vi "Identify Contraction Segment.vi"(10 "Intra-cursor segment":dynamicdata(waveform), 11 "Contraction Onset":dbl) -> (1 "Con Ons on I-C Segment":dbl, 2 "Contraction Segment":dynamicdata(waveform), 3 "Con Ons Segment":dynamicdata(waveform), 4 "trigger location":dbl)   [LabVIEW 2016]
uses:
  <vilib>/measure/mamon.llb/Trigger Detection for 1 Channel.vi
  <vilib>/measure/NI_MAPro.lvlib
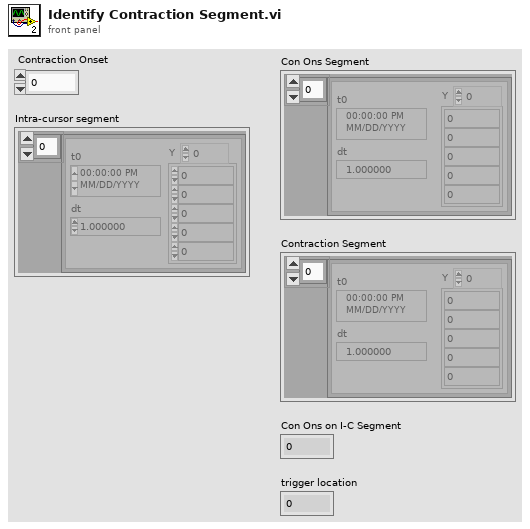
[diagram p1: front panel]
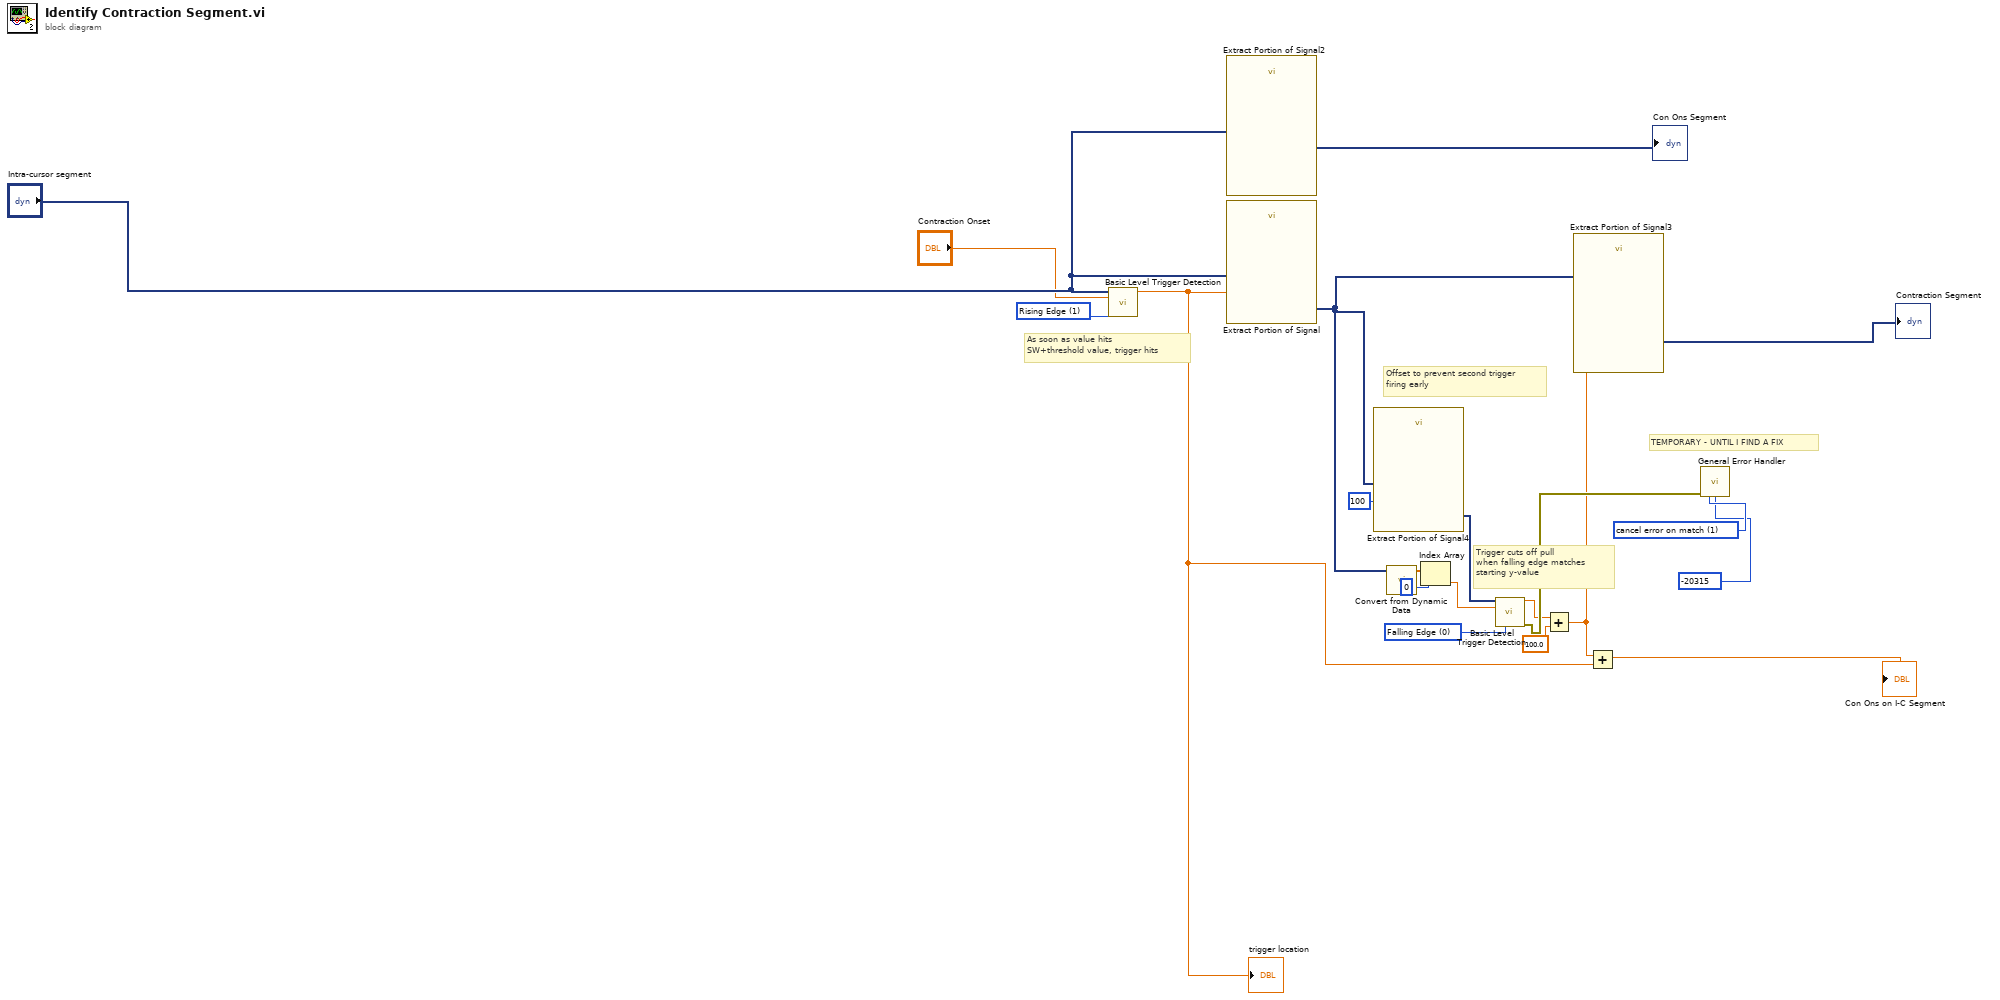
[diagram p0: block diagram]
diagram:
  w19 = 1 items=["no exception", "cancel error on match", "set error on match"] ("[exception action] (none:0)")
  w3 = u16 0 items=["Falling Edge", "Rising Edge"] ("trigger slope")
  w1 = u16 1 items=["Falling Edge", "Rising Edge"] ("trigger slope")
  # "TEMPORARY - UNTIL I FIND A FIX"
  # "Offset to prevent second trigger\nfiring early"
  # "Trigger cuts off pull\nwhen falling edge matches \nstarting y-value"
  # "As soon as value hits \nSW+threshold value, trigger hits"
  n1 = call-poly <vilib>:"Basic Level Trigger Detection.vi"("signal in"="Intra-cursor segment", "level"="Contraction Onset", "trigger slope"=w1) -> ("trigger location"=w11:dbl)  [unwired: 10 in, 2 out]
  "trigger location" <- w11
  n2 = call "Extract Portion of Signal2"("Signals"="Intra-cursor segment") -> ("Section"=→"Con Ons Segment":dynamicdata)  [unwired: 9 in, 1 out]
  n3 = call "Extract Portion of Signal"("Begin Sample"=w11, "Signals"="Intra-cursor segment") -> ("Section"=w12:dynamicdata)  [unwired: 8 in, 1 out]
  n4 = call "Extract Portion of Signal4"("Begin Sample"=100, "Signals"=w12) -> ("Section"=w14:dynamicdata)  [unwired: 8 in, 1 out]
  n5 = call "Convert from Dynamic Data"("Dynamic Data Type"=w12) -> ("Array"=w7:dbl[])  [unwired: 3 in]
  n6 = Index Array(array=w7, index=0) -> (element=w9:dbl)
  n7 = call-poly <vilib>:"Basic Level Trigger Detection.vi"("signal in"=w14, "level"=w9, "trigger slope"=w3) -> ("trigger location"=w16:dbl, "error out"=w20:errorcluster)  [unwired: 10 in, 1 out]
  n8 = Add(x=w16, y=100.0) -> (x+y=w15:dbl)
  n9 = call "Extract Portion of Signal3"("Samples"=w15, "Signals"=w12) -> ("Section"=→"Contraction Segment":dynamicdata)  [unwired: 8 in, 1 out]
  n10 = Add(x=w15, y=w11) -> (x+y=→"Con Ons on I-C Segment":dbl)
  n11 = call <vilib>:"General Error Handler.vi"("error in (no error)"=w20, "[exception action] (none:0)"=w19, "[exception code]"=-20315 ("error code (no error:0)")) -> ()  [unwired: 8 in, 5 out]
